vi "BenchC2_DEV_v15_5.vi"() -> ()   [LabVIEW 2017]
uses:
  x64/Debug/BERTTA.dll
panel:
  out "Started:":string
  in  "SHUTDOWN":bool
  in  "MASTER CONTROL":bool
  in  "Tab Control":T1(tab)
  out "Output File":path caption="selected path"
  in  "Browse folder":path=path "" caption="start path"
  in  "Read Seq":bool
  in  "Save Seq":bool
  in  "Configuration file":path caption="Filename"
  in  "OK Button 2":bool
  out "Boolean":bool
  in  "User (initials)":string
  in  "Project name":string
  in  "Description":string
  out "Led11 12":bool
  out "Led11 11":bool
  out "PUMP1":bool
  out "Target amount":dbl format="Target amount:        %#_g"
  out "Scale weight":dbl format="Scale weight:     %#_4g"
  out "Amount now":dbl format="Amount now:      %#_4g"
  out "Flow rate":dbl format="Flow rate:                   %#_4g"
  out "Time to target":dbl format="Time to target:     %<%H:%M:%S>t"
  out "Current step":dbl format="Current step:              %#_g"
  out "Target":dbl format="Target:                %#_4g"
  out "Amount now":dbl format="Amount now:    %#_4g"
  out "Amount now":dbl
  out "Target":dbl
  out "Current step":dbl
  out "Time to target":dbl format="%<%H:%M:%S>t"
  out "Flow rate":dbl
  out "Amount now":dbl
  out "Scale weight":dbl
  out "Target amount":dbl
  out "PUMP2":bool
  out "Sensor OK 6":bool
  out "Sensor OK 5":bool
  out "Sensor OK 4":bool
  out "Sensor OK 3":bool
  in  "OK Button":bool
  in  "Add comment":string
  out "Tr":dbl format="Tr:              %#_4g"
  out "Tj in":dbl format="Tj in:        %#_4g"
  out "Tj out":dbl format="Tj out:        %#_4g"
  out "T set":dbl format="T set:          %#_g"
  out "Current step":i32 format="Current step:  %.0f"
  out "RPM":dbl format="RPM:          %#_g"
  out "Torque 2":dbl format="Torque:      %#_g"
  out "PUMP3":bool
  out "Target amount":dbl
  out "Scale weight":dbl
  out "Amount now":dbl
  out "Flow rate":dbl
  out "Time to target":dbl format="%<%H:%M:%S>t"
  out "Current step":dbl
  out "Target":dbl
  out "Amount now":dbl
  out "Waveform Chart 5":dynamicdata(graph)
  out "Waveform Chart 6":dynamicdata(graph)
  out "Waveform Chart 7":dynamicdata(graph)
  out "Led11 10":bool
  out "T external 3":dbl format="T (S2):       %#_4g"
  out "Table":string[][](table)=[["14.8.2017 18.06.59", "0,000000", "417,670000", "-0,150000", "1,000000", "22,220000", "23,366837", "23,574959", "23,985852", "23,690000", "240,000000", "4,000000", "0,000000", "397,000000", "-397,000000", "1,000000"], ["14.8.2017 18.07.06", "0,000000", "417,640000", "-0,120000", "1,000000", "22,220000", "23,763115", "23,906257", "23,985694", "23,680000", "240,000000", "4,000000", "0,000000", "397,000000", "-397,000000", "1,000000"], ["14.8.2017 18.07.13", "0,000000", "417,640000", "-0,120000", "1,000000", "22,220000", "23,965922", "24,013440", "23,984906", "23,670000", "240,000000", "4,100000", "3,000000", "397,000000", "-397,000000", "1,000000"], ["14.8.2017 18.07.21", "0,000000", "417,640000", "-0,120000", "1,000000", "22,220000", "23,943860", "23,900110", "23,987113", "23,670000", "240,000000", "4,000000", "0,000000", "397,000000", "-397,000000", "1,000000"], ["14.8.2017 18.07.28", "0,000000", "417,640000", "-0,120000", "1,000000", "22,220000", "23,736328", "23,600018", "23,989004", "23,660000", "240,000000", "4,000000", "0,000000", "397,000000", "-397,000000", "1,000000"], ["14.8.2017 18.07.36", "0,000000", "417,640000", "-0,120000", "1,000000", "22,220000", "23,480910", "23,324538", "23,991053", "23,660000", "240,000000", "4,000000", "0,000000", "397,000000", "-397,000000", "1,000000"], ["14.8.2017 18.07.43", "0,000000", "417,640000", "-0,120000", "2,000000", "22,220000", "23,195579", "23,008270", "23,999093", "23,650000", "240,000000", "4,000000", "0,000000", "397,000000", "-397,000000", "1,000000"], ["14.8.2017 18.07.51", "0,000000", "417,650000", "-417,650000", "1,000000", "22,220000", "22,862541", "22,649021", "24,003979", "23,650000", "240,000000", "4,000000", "0,000000", "397,000000", "-397,000000", "2,000000"], ["14.8.2017 18.07.58", "0,000000", "417,640000", "0,010000", "1,000000", "22,220000", "22,541353", "22,354878", "24,005398", "23,650000", "240,000000", "4,000000", "0,000000", "397,000000", "-397,000000", "1,000000"], ["14.8.2017 18.08.06", "0,000000", "417,640000", "0,010000", "1,000000", "22,220000", "22,347931", "22,253738", "24,007605", "23,640000", "240,000000", "4,100000", "0,000000", "397,000000", "-397,000000", "1,000000"], ["14.8.2017 18.08.13", "0,000000", "417,640000", "0,010000", "1,000000", "22,220000", "22,329030", "22,302102", "24,006028", "23,640000", "240,000000", "4,000000", "0,000000", "395,820000", "-395,820000", "1,000000"], ["14.8.2017 18.08.20", "0,000000", "417,640000", "0,010000", "1,000000", "22,220000", "22,466849", "22,511320", "24,002403", "23,630000", "240,000000", "4,000000", "0,000000", "395,830000", "-0,010000", "1,000000"], ["14.8.2017 18.08.28", "0,000000", "417,640000", "0,010000", "1,000000", "22,220000", "22,707062", "22,835101", "24,000984", "23,620000", "240,000000", "4,000000", "0,000000", "395,830000", "-0,010000", "1,000000"], ["14.8.2017 18.08.35", "0,000000", "417,640000", "0,010000", "1,000000", "22,220000", "23,054104", "23,232979", "24,001299", "23,600000", "240,000000", "4,000000", "0,000000", "395,830000", "-0,010000", "1,000000"], ["14.8.2017 18.08.43", "0,000000", "417,640000", "0,010000", "1,000000", "22,220000", "23,412371", "23,522793", "24,002560", "23,590000", "240,000000", "4,000000", "0,000000", "395,820000", "0,000000", "1,000000"], ["14.8.2017 18.08.51", "0,000000", "417,640000", "0,010000", "1,000000", "22,220000", "23,596247", "23,656125", "24,003821", "23,580000", "240,000000", "4,000000", "0,000000", "395,820000", "0,000000", "1,000000"]]
  out "LED_5":bool
  out "LED_4":bool
  in  "PAUSE/RUN 4":bool
  in  "TEMP RAMP":dbl[][](array[numeric])
  out "LED_3":bool
  out "LED_2":bool
  out "LED_1":bool
  out "LED_MANUAL":bool
  in  "Reset 6":bool
  in  "Manual/Ramp":bool=TRUE
  in  "Sensor selector":bool=TRUE
  in  "Tr/Tj mode selector":bool=TRUE
  out "LED STOP":bool
  in  "Failsafe":dbl=20.0 format="Failsafe temperature:            %#_g"
  out "Current temp":dbl format="Current temperature S1:       %#_4g"
  out "Sensor OK":bool
  out "T external 2":dbl format="Current temperature S2:       %#_4g"
  in  "OK Button 3":bool
  out "Waveform Chart":dynamicdata(graph)
  in  "X scale":i64(slide)=50 scale=0.0..100.0
  out "Led11 7":bool
  out "Led11 6":bool
  out "Led11 7":bool
  out "Led11 6":bool
  out "Led5 7":bool
  out "Led4 6":bool
  out "Waveform Chart 18":dynamicdata(graph)
  in  "PAUSE/RUN 3":bool
  in  "Tube select 3":u32(ring) items=["Big tube", "Double big tube", "Medium tube", "Small tube"]
  in  "Reset 8":bool
  out "Led11 9":bool
  in  "?":bool
  in  "Grams / min 3":dbl
  out "RPM 3":dbl format="%_4f"
  out "Flow rate (g/min) 3":dbl
  out "Scale reading 3":dbl
  out "Step amount now 3":dbl
  out "Total amount now 3":dbl
  out "Elapsed / step 3":dbl format="%<%H:%M:%S>t"
  out "Time to target 3":dbl format="%<%H:%M:%S>t"
  out "Led5 5":bool
  out "Led4 5":bool
  out "Led3 5":bool
  out "Led2 5":bool
  out "Led1 5":bool
  in  "PumpSeq 6":dbl[][](array[numeric])=[[0.0, 0.0, 0.0, 0.0, 0.0, 0.0, 0.0, 0.0, 0.0, 0.0], [0.0, 0.0, 0.0, 0.0, 0.0, 0.0, 0.0, 0.0, 0.0, 0.0], [0.0, 0.0, 0.0, 0.0, 0.0, 0.0, 0.0, 0.0, 0.0, 0.0], [0.0, 0.0, 0.0, 0.0, 0.0, 0.0, 0.0, 0.0, 0.0, 0.0], [0.0, 0.0, 0.0, 0.0, 0.0, 0.0, 0.0, 0.0, 0.0, 0.0], [0.0, 0.0, 0.0, 0.0, 0.0, 0.0, 0.0, 0.0, 0.0, 0.0], [0.0, 0.0, 0.0, 0.0, 0.0, 0.0, 0.0, 0.0, 0.0, 0.0], [0.0, 0.0, 0.0, 0.0, 0.0, 0.0, 0.0, 0.0, 0.0, 0.0], [0.0, 0.0, 0.0, 0.0, 0.0, 0.0, 0.0, 0.0, 0.0, 0.0], [0.0, 0.0, 0.0, 0.0, 0.0, 0.0, 0.0, 0.0, 0.0, 0.0]]
  out "Led11 8":bool
  in  "PAUSE/RUN 2":bool
  in  "Tube select 2":u32(ring) items=["Big tube", "Double big tube", "Medium tube", "Small tube"]
  out "Led11 7":bool
  in  "?":bool
  in  "Grams / min 2":dbl
  out "RPM 2":dbl format="%_4f"
  out "Flow rate (g/min) 2":dbl
  out "Scale reading 2":dbl
  out "Step amount now 2":dbl
  out "Total amount now 2":dbl
  out "Elapsed / step 2":dbl format="%<%H:%M:%S>t"
  out "Time to target 2":dbl format="%<%H:%M:%S>t"
  out "Led5 4":bool
  out "Led4 4":bool
  out "Led3 4":bool
  out "Led2 4":bool
  out "Led1 4":bool
  in  "PumpSeq 5":dbl[][](array[numeric])=[[0.0, 0.0, 0.0, 0.0, 0.0, 0.0, 0.0, 0.0, 0.0, 0.0], [0.0, 0.0, 0.0, 0.0, 0.0, 0.0, 0.0, 0.0, 0.0, 0.0], [0.0, 0.0, 0.0, 0.0, 0.0, 0.0, 0.0, 0.0, 0.0, 0.0], [0.0, 0.0, 0.0, 0.0, 0.0, 0.0, 0.0, 0.0, 0.0, 0.0], [0.0, 0.0, 0.0, 0.0, 0.0, 0.0, 0.0, 0.0, 0.0, 0.0], [0.0, 0.0, 0.0, 0.0, 0.0, 0.0, 0.0, 0.0, 0.0, 0.0], [0.0, 0.0, 0.0, 0.0, 0.0, 0.0, 0.0, 0.0, 0.0, 0.0], [0.0, 0.0, 0.0, 0.0, 0.0, 0.0, 0.0, 0.0, 0.0, 0.0], [0.0, 0.0, 0.0, 0.0, 0.0, 0.0, 0.0, 0.0, 0.0, 0.0], [0.0, 0.0, 0.0, 0.0, 0.0, 0.0, 0.0, 0.0, 0.0, 0.0]]
  out "Led11 6":bool
  in  "Reset 7":bool
  in  "PAUSE/RUN":bool
  in  "Tube select":u32(ring) items=["Big tube", "Double big tube", "Medium tube", "Small tube"]
  out "Led11 5":bool
  out "RPM":dbl format="RPM                      %_4f"
  out "Flow rate (g/min)":dbl format="Flow rate               %#_g"
  out "Scale reading":dbl format="Scale reading       %#_g"
  out "Step amount now":dbl format="Step amount       %#_g"
  out "Total amount now":dbl format="Total amount      %#_g"
  out "Elapsed / step":dbl format="Elapsed / step      %<%H:%M:%S>t"
  out "Time to target":dbl format="Time to target     %<%H:%M:%S>t"
  out "Led5 3":bool
  out "Led4 3":bool
  out "Led3 3":bool
  out "Led2 3":bool
  out "Led1 3":bool
  in  "PumpSeq 4":dbl[][](array[numeric])=[[0.0, 0.0, 0.0, 0.0, 0.0, 0.0, 0.0, 0.0, 0.0, 0.0], [0.0, 0.0, 0.0, 0.0, 0.0, 0.0, 0.0, 0.0, 0.0, 0.0], [0.0, 0.0, 0.0, 0.0, 0.0, 0.0, 0.0, 0.0, 0.0, 0.0], [0.0, 0.0, 0.0, 0.0, 0.0, 0.0, 0.0, 0.0, 0.0, 0.0], [0.0, 0.0, 0.0, 0.0, 0.0, 0.0, 0.0, 0.0, 0.0, 0.0], [0.0, 0.0, 0.0, 0.0, 0.0, 0.0, 0.0, 0.0, 0.0, 0.0], [0.0, 0.0, 0.0, 0.0, 0.0, 0.0, 0.0, 0.0, 0.0, 0.0], [0.0, 0.0, 0.0, 0.0, 0.0, 0.0, 0.0, 0.0, 0.0, 0.0], [0.0, 0.0, 0.0, 0.0, 0.0, 0.0, 0.0, 0.0, 0.0, 0.0], [0.0, 0.0, 0.0, 0.0, 0.0, 0.0, 0.0, 0.0, 0.0, 0.0]]
  in  "?":bool
  in  "Grams / min":dbl format="Manual g/min:  %#_g"
  out "Led11 4":bool
  in  "Reset 5":bool
  in  "OK Button 4":bool
  out "Waveform Chart 16":dynamicdata(graph)
  in  "OK Button 5":bool
  out "Waveform Chart 17":dynamicdata(graph)
  in  "OK Button 6":bool
  in  "PAUSE/RUN 5":bool
  in  "?":bool
  in  "Scale port":dbl=5.0
  out "Waveform Chart 15":dynamicdata(graph)
  in  "OK Button 8":bool
  in  "PAUSE/RUN 6":bool
  in  "Set RPM":i32
  in  "Remote / Manual":bool
  out "RPM":dbl
  out "Torque":dbl
  out "Waveform Chart 4":dynamicdata(graph)
  in  "OK Button 7":bool
  in  "CDAQ Temp Control":tag="cDAQ9188XT-1C3BF12Mod1"
  in  "CDAQ PAM Control":tag="cDAQ9188XT-1C3BF12Mod1"
  in  "PORT PUMP2":i32 format="PUMP 2 PORT:  %.0f"
  in  "PORT PUMP3":i32 format="PUMP 3 PORT:  %.0f"
  in  "PORT PUMP1":i32 format="PUMP 1 PORT:  %.0f"
  in  "Save PortDev":bool
  in  "LAUDA":i32 format="LAUDA PORT:  %.0f"
  in  "HEIDOLPH":i32 format="HEIDOLPH PORT:  %.0f"
  in  "SCALE1":i32 format="SCALE 1 PORT:  %.0f"
  in  "SCALE2":i32 format="SCALE 2 PORT:  %.0f"
  in  "SCALE 3":i32 format="SCALE 3 PORT:  %.0f"
  # "PUMP & SCALE 1"
  # "PUMP & SCALE 2"
  # "PUMP & SCALE 3"
  # "STEP"
  # "STEP"
  # "STEP"
  # "TOTAL"
  # "TOTAL"
  # "TOTAL"
  # "Temperature sensor:"
  # "Manual control:"
  # "MANUAL"
  # "RAMP"
  # "Temp Target       Time Target          Wait Time"
  # "STOP"
  # "g              min"
  # "g              min"
  # "g              min"
  # "PAM control"
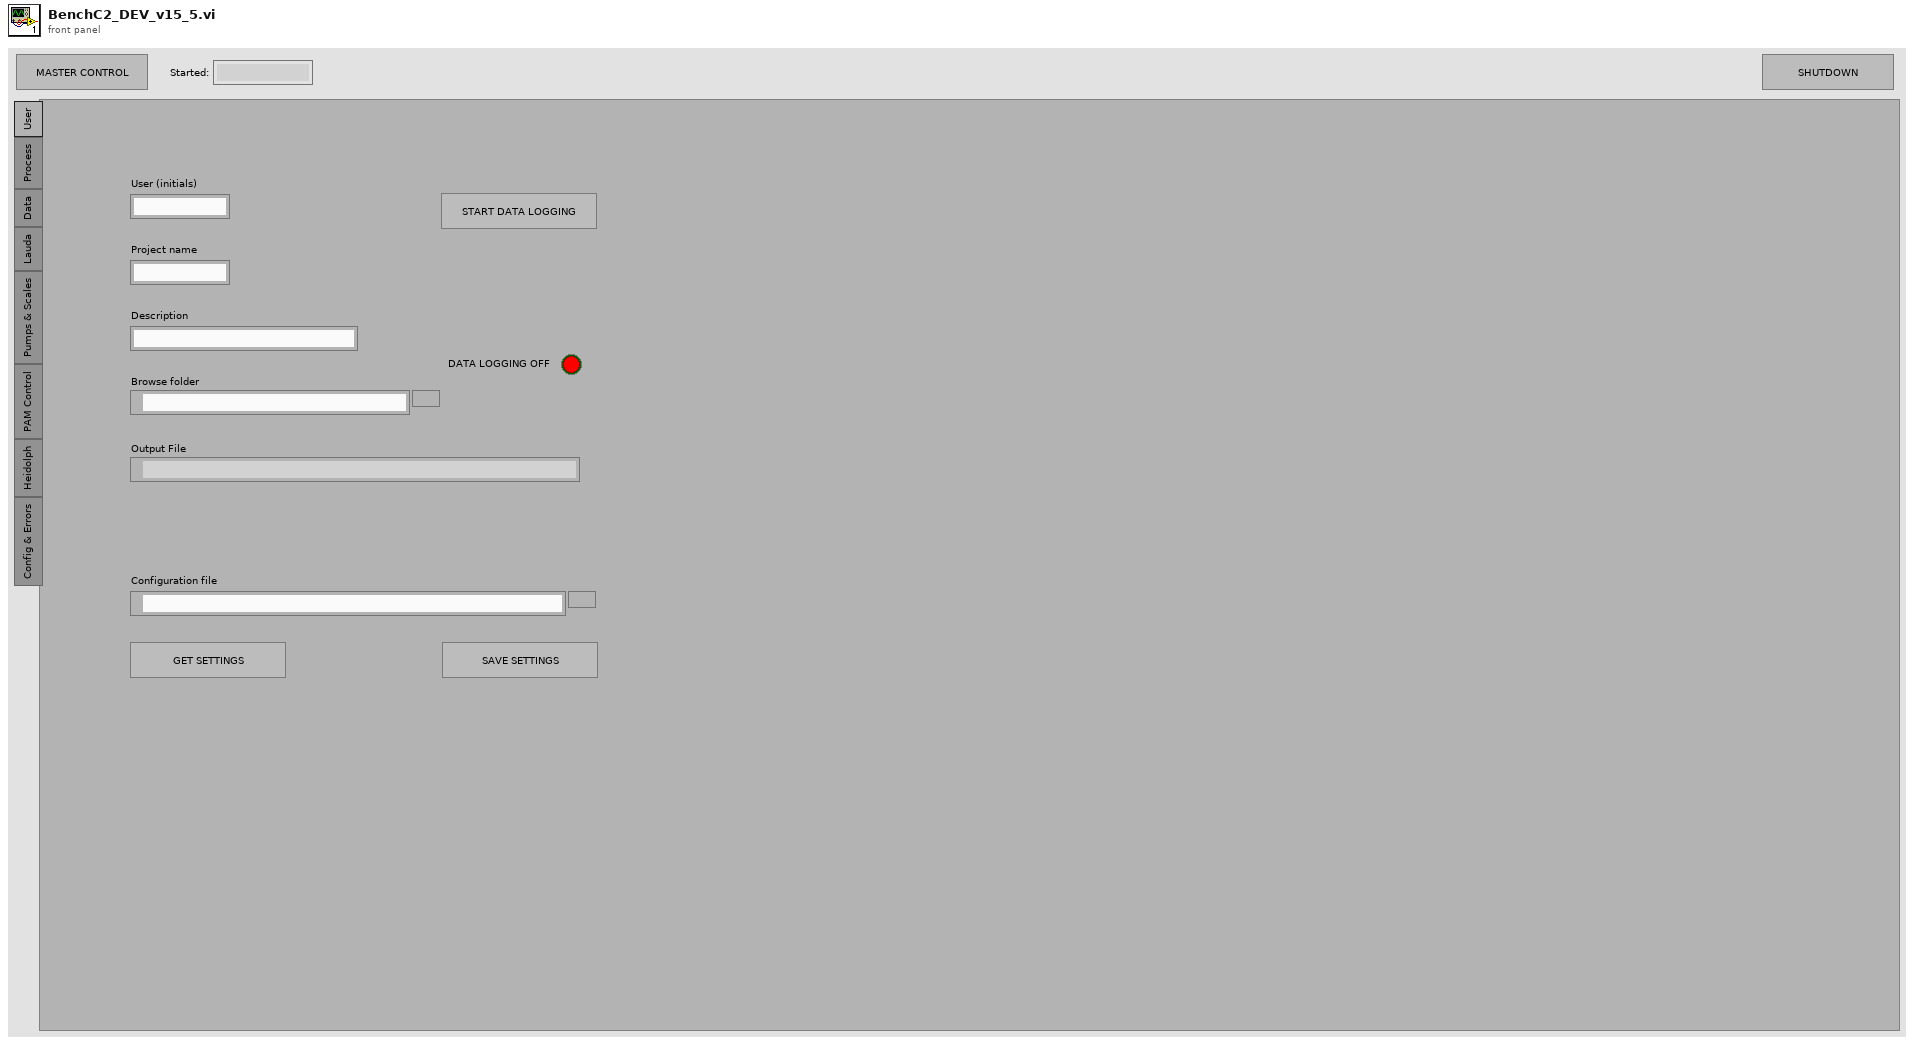
[diagram p1: front panel]
types:
  T1 = enum32{"User", "Process", "Data", "Lauda", "Pumps & Scales", "PAM Control", "Heidolph", "Config & Errors"}
diagram:
  n1 = while {
    i -> [w217]
    stop <- FALSE stop-if-true
    w49 = i64 1000 ("y")
    # "TARKISTA: negatiiviset lämpötilat, toimivatko"
    # "X-skaalaus puuttuu"
    # "SCALE & PUMP 1"
    # "SCALE & PUMP 3"
    n2 = And(x="PAUSE/RUN 6", y="MASTER CONTROL") -> (x .and. y?=w30:bool)
    n3 = feedback #1() -> (w54:dbl[][])  [unwired: 1 in]
    n4 = Select(t="TEMP RAMP", s="Reset 6", f=w54) -> (s? t:f=w55:dbl[][])
    n5 = feedback-in #1(w55) -> ()
    n6 = Initialize Array(0.0 ("element"), 5 ("dimension size"), 3 ("dimension size")) -> (w98:dbl[][])
    n7 = Select(t="Set RPM", s=w30, f=10) -> (s? t:f=w33:i32)
    n8 = Not(x="MASTER CONTROL") -> (.not. x?=w266:bool)
    n9 = Replace Array Subset(array=w98, new element=w54, index (row)=0, index (col)=0 ("disabled index (col)")) -> (w72:dbl[][])
    n10 = control-ref of="This VI"() -> (w26:refnum<vi>)
    n11 = Multiply(x="X scale", y=w49) -> (x*y=w50:i64)
    n12 = Boolean To (0,1)(Boolean=w266) -> (0, 1=w267:i16)
    n13 = Add(x=w50, y=w49) -> (x+y=w45:i64)
    n14 = for {
      N: w267 -> [_]
      n15 = Get Date/Time String(want seconds? (F)=TRUE) -> (time string=→"Started:":string)  [unwired: 2 in, 1 out]
    }
    n16 = feedback #2() -> (w48:i64)  [unwired: 1 in]
    n17 = feedback-in #2(w45) -> ()
    n18 = Boolean To (0,1)(Boolean="Sensor selector") -> (0, 1=w80:i16)
    n19 = Boolean To (0,1)(Boolean="SHUTDOWN") -> (0, 1=w24:i16)
    n20 = call "shutdown sequence.vi"("SHUTDOWN"="SHUTDOWN", "VI in"=w26) -> ()  [unwired: 10 in]
    n21 = Not Equal?(x=w48, y=w45) -> (x != y?=w47:bool)
    n22 = property on="Waveform Chart" class="WFChart (strict)"() -> ("History Data"=w52:dynamicdata[])  [unwired: 2 in, 2 out]
    n23 = Boolean To (0,1)(Boolean=w47) -> (0, 1=w44:i16)
    n24 = Array Size(array=w52) -> (size(s)=w46:i32)
    n25 = Boolean To (0,1)(Boolean="SHUTDOWN") -> (0, 1=w27:i16)
    n26 = Boolean To (0,1)(Boolean="Tr/Tj mode selector") -> (0, 1=w92:i16)
    n27 = formula code="int SensorLED1 = 0, SensorLED0 = 0, ModeLED1 = 0, ModeLED0 = 0;\nif(Sensor==1) SensorLED1 = 1;\nif(Sensor==0) SensorLED0 = 1;\nif(Tr_Tj==1) ModeLED1 = 1;\nif(Tr_Tj==0) ModeLED0 = 1;"("Tr_Tj"=w92, "Sensor"=w80) -> ("SensorLED1"=w90:i32, "SensorLED0"=w88:i32, "ModeLED1"=w73:i32, "ModeLED0"=w83:i32)
    n28 = Equal?(x=w90, y=1.0) -> (x = y?=→"Sensor OK 3":bool)
    n29 = Equal?(x=w88, y=1.0) -> (x = y?=→"Sensor OK 4":bool)
    n30 = for {
      N: w44 -> [_]
      tunnel: w46 -> [w274]
      tunnel: w45 -> [w273]
      n31 = Add(x=w274, y=w273) -> (x+y=w272:i64)
      n32 = property on="Waveform Chart" class="WFChart (strict)"("XScale.Maximum"=w272) -> ()  [unwired: 2 in, 2 out]
    }
    n33 = call "MReadRS232_2.vi"("port1"="LAUDA", "dev1"=1, "port2"="LAUDA", "dev2"=2, "port3"="HEIDOLPH", "dev7"=5, "dev8"=0, "port7"="SCALE 3", "port8"=0, "dev5"=5, "port5"="SCALE1", "dev4"=4, "dev6"=5, "port6"="SCALE2", "port4"="HEIDOLPH", "dev3"=3) -> ("params"=w1:dbl[])  [unwired: 2 in, 1 out]
    n34 = call "HEI_CTRL.vi"("shutdown"=w27, "Set RPM"=w33, "Remote / Manual"="Remote / Manual", "port3"="HEIDOLPH") -> ()  [unwired: 8 in]
    n35 = And(x="MASTER CONTROL", y="PAUSE/RUN 4") -> (x .and. y?=w116:bool)
    n36 = Index Array(array=w72, index (col)=2 ("disabled index (col)")) -> (element=w104:dbl[])  [unwired: 1 in]
    n37 = Equal?(x=w73, y=1.0) -> (x = y?=→"Sensor OK 6":bool)
    n38 = Equal?(x=w83, y=1.0) -> (x = y?=→"Sensor OK 5":bool)
    n39 = Boolean To (0,1)(Boolean=w116) -> (0, 1=w115:i16)
    n40 = Boolean To (0,1)(Boolean="Manual/Ramp") -> (0, 1=w117:i16)
    n41 = Boolean To (0,1)(Boolean="Reset 6") -> (0, 1=w119:i16)
    n42 = Build Array("LAUDA", "HEIDOLPH", "SCALE1", "SCALE2", "SCALE 3", "PORT PUMP1", "PORT PUMP2", "PORT PUMP3") -> (w59:i32[])
    n43 = Index Array(array=w72, index (col)=1 ("disabled index (col)")) -> (element=w106:dbl[])  [unwired: 1 in]
    n44 = Index Array(array=w72, index (col)=0 ("disabled index (col)")) -> (element=w107:dbl[])  [unwired: 1 in]
    n45 = call "LaudaDAQ.vi"("device name"="CDAQ Temp Control") -> (1:"Tj out"=→"Tj out":dbl, "data"=w254:dynamicdata, "Sensor OK"=→"Sensor OK":bool, 4:"Tj out"=→"Tj in":dbl, "T external 2"=w29:dbl)  [unwired: 5 in, 1 out]
    "T external 2" <- w29
    "T external 3" <- w29
    n46 = call "Ramp_Lauda_v3.vi"("manual"=w117, "Tr_Tj"=w92, "shutdown"=w24, "S1_S2"=w80, "Tr"=w1, "T_fail"="Failsafe", "enable"=w115, "time_set"=w106, "reset"=w119, "time_wait"=w104, "T_S2"=w29, "port"="LAUDA", "T_sp"=w107) -> ("LED_1"=→"LED_1":bool, "LED_manual"=→"LED_MANUAL":bool, "LED_2"=→"LED_2":bool, "step"=w70:dbl, "LED_stop"=→"LED STOP":bool, "LED_3"=→"LED_3":bool, "LED 4"=→"LED_4":bool, "LED 5"=→"LED_5":bool, "setpoint"=w67:dbl, "Tr_out"=w114:dbl, "T int"=w113:dbl)  [unwired: 2 in, 2 out]
    "Tr" <- w114
    "T set" <- w67
    "Current temp" <- w114
    n47 = Boolean To (0,1)(Boolean="Save PortDev") -> (0, 1=w220:i16)
    n48 = for {
      N: w220 -> [_]
      tunnel: w59 -> [w320]
      tunnel: "Save PortDev" -> [w321]
      n49 = call "Convert to Dynamic Data"("Array"=w320) -> ("Dynamic Data Type"=w319:dynamicdata)  [unwired: 3 in]
      n50 = call "Write To Measurement File3"("Signals"=w319, "Reset"=w321) -> ()  [unwired: 15 in, 3 out]
    }
    n51 = Add(x=w70, y=1.0) -> (x+y=→"Current step":dbl)
    n52 = Less?(x=w217, y=1.0) -> (x < y?=w215:bool)
    n53 = Index Array(array=w1, index=3) -> (element=w208:dbl)
    "RPM" <- w208
    "RPM" <- w208
    n54 = Index Array(array=w1, index=2) -> (element=w210:dbl)
    n55 = Boolean To (0,1)(Boolean=w215) -> (0, 1=w216:i16)
    n56 = Divide(x=w210, y=10.0) -> (x/y=w207:dbl)
    "Torque" <- w207
    "Torque 2" <- w207
    n57 = for {
      N: w216 -> [_]
      tunnel: w215 -> [w314]
      n58 = while {
        tunnel: [w317] -> w313
        tunnel: w314 -> [w315]
        stop <- w318 stop-if-true
        n59 = call "Read From Measurement File2"("Enable"=TRUE, "Reset"=w315) -> ("Signals"=w317:dynamicdata, "EOF?"=w318:bool)  [unwired: 4 in, 4 out]
      }
      n60 = call "Convert from Dynamic Data2"("Dynamic Data Type"=w313) -> ("Array"=w299:dbl[])  [unwired: 3 in]
      n61 = Index Array(array=w299, index=0) -> (element=w306:dbl)
      n62 = Index Array(array=w299, index=1) -> (element=w305:dbl)
      n63 = Index Array(array=w299, index=2) -> (element=w304:dbl)
      n64 = Index Array(array=w299, index=3) -> (element=w303:dbl)
      n65 = Index Array(array=w299, index=4) -> (element=w302:dbl)
      n66 = Index Array(array=w299, index=5) -> (element=w296:dbl)
      n67 = Index Array(array=w299, index=6) -> (element=w298:dbl)
      n68 = Index Array(array=w299, index=7) -> (element=w297:dbl)
      n69 = property on="LAUDA" class="DigNum (strict)"("Val(Sgnl)"=w306) -> ()  [unwired: 2 in, 2 out]
      n70 = property on="HEIDOLPH" class="DigNum (strict)"("Val(Sgnl)"=w305) -> ()  [unwired: 2 in, 2 out]
      n71 = property on="SCALE1" class="DigNum (strict)"("Val(Sgnl)"=w304) -> ()  [unwired: 2 in, 2 out]
      n72 = property on="SCALE2" class="DigNum (strict)"("Val(Sgnl)"=w303) -> ()  [unwired: 2 in, 2 out]
      n73 = property on="SCALE 3" class="DigNum (strict)"("Val(Sgnl)"=w302) -> ()  [unwired: 2 in, 2 out]
      n74 = property on="PORT PUMP2" class="DigNum (strict)"("Val(Sgnl)"=w298) -> ()  [unwired: 2 in, 2 out]
      n75 = property on="PORT PUMP3" class="DigNum (strict)"("Val(Sgnl)"=w297) -> ()  [unwired: 2 in, 2 out]
      n76 = property on="PORT PUMP1" class="DigNum (strict)"("Val(Sgnl)"=w296) -> ()  [unwired: 2 in, 2 out]
    }
    n77 = Merge Signals(w208, w207) -> (w206:dynamicdata)
    "Waveform Chart 4" <- w206
    "Waveform Chart 6" <- w206
    n78 = Boolean To (0,1)(Boolean="OK Button 3") -> (0, 1=w235:i16)
    n79 = for {
      N: w235 -> [_]
      n80 = property on="Waveform Chart" class="WFChart (strict)"("History Data"=dynamicdata[] []) -> ()  [unwired: 2 in, 2 out]
    }
    n81 = Merge Signals(w67, w114, w113, w254) -> (w255:dynamicdata)
    "Waveform Chart" <- w255
    "Waveform Chart 5" <- w255
    n82 = Boolean To (0,1)(Boolean="OK Button 4") -> (0, 1=w233:i16)
    n83 = for {
      N: w233 -> [_]
      n84 = property on="Waveform Chart 18" class="WFChart (strict)"("History Data"=dynamicdata[] []) -> ()  [unwired: 2 in, 2 out]
    }
    n85 = Boolean To (0,1)(Boolean="OK Button 5") -> (0, 1=w78:i16)
    n86 = call "IsmaCTRL.vi"("FR_manual"="Grams / min", "Manual"="?", "Reset"="Reset 5", "Pause"="PAUSE/RUN", "Setpoint_W   /   Setpoint_T"="PumpSeq 4", "Enable"="MASTER CONTROL", "Scale"=w1) -> ("Boolean 9"=→"Led11 5" →"Led11 10":bool, "Boolean"=→"Led1 3":bool, "Boolean 2"=→"Led2 3":bool, "Boolean 3"=→"Led3 3":bool, "Boolean 4"=→"Led4 3":bool, "Boolean 5"=→"Led5 3":bool, "Boolean 6"=→"Led4 6":bool, "Boolean 7"=→"Led5 7":bool, "FR"=w6:dbl, "RPM"=w5:dbl, "Weight"=w4:dbl, "elapsed"=→"Elapsed / step":dbl, "time_to_target"=→"Time to target" →"Time to target":dbl, "pumpCTRL"=w18:dbl, "Boolean 8"=w10:bool)  [unwired: 6 in]
    "Flow rate" <- w6
    "Scale weight" <- w4
    "Led11 4" <- w10
    "Scale reading" <- w4
    "Flow rate (g/min)" <- w6
    "RPM" <- w5
    n87 = for {
      N: w78 -> [_]
      n88 = property on="Waveform Chart 16" class="WFChart (strict)"("History Data"=dynamicdata[] []) -> ()  [unwired: 2 in, 2 out]
    }
    n89 = Greater?(x=w18, y=70.0) -> (0:→"PUMP1":bool)
    n90 = Merge Signals(w4, w6) -> (w79:dynamicdata)
    "Waveform Chart 18" <- w79
    n91 = Multiply(x=-1.0, y=w4) -> (x*y=→"Amount now" →"Total amount now":dbl)
    n92 = Boolean To (0,1)(Boolean="OK Button 6") -> (0, 1=w76:i16)
    n93 = for {
      N: w76 -> [_]
      n94 = property on="Waveform Chart 17" class="WFChart (strict)"("History Data"=dynamicdata[] []) -> ()  [unwired: 2 in, 2 out]
    }
    n95 = And(x="PAUSE/RUN", y=w10) -> (x .and. y?=w194:bool)
    n96 = feedback #3() -> (w195:bool)  [unwired: 1 in]
    n97 = feedback-in #3(w194) -> ()
    n98 = Not Equal?(x=w195, y=w194) -> (x != y?=w193:bool)
    n99 = Boolean To (0,1)(Boolean=w193) -> (0, 1=w192:i16)
    n100 = for {
      N: w192 -> [_]
      n101 = property on="PAUSE/RUN" class="Bool (strict)"("Val(Sgnl)"=FALSE ("Value (Signaling)")) -> ()  [unwired: 2 in, 2 out]
    }
    n102 = Boolean To (0,1)(Boolean="OK Button 7") -> (0, 1=w231:i16)
    n103 = for {
      N: w231 -> [_]
      n104 = property on="Waveform Chart 4" class="WFChart (strict)"("History Data"=dynamicdata[] []) -> ()  [unwired: 2 in, 2 out]
    }
    n105 = Boolean To (0,1)(Boolean="OK Button 8") -> (0, 1=w203:i16)
    n106 = for {
      N: w203 -> [_]
      n107 = property on="Waveform Chart 15" class="WFChart (strict)"("History Data"=dynamicdata[] []) -> ()  [unwired: 2 in, 2 out]
    }
    n108 = Index Array(array="PumpSeq 5", index (col)=0) -> (element=w175:dbl[])  [unwired: 1 in]
    n109 = Index Array(array="PumpSeq 5", index (col)=1) -> (element=w176:dbl[])  [unwired: 1 in]
    n110 = Boolean To (0,1)(Boolean="PAUSE/RUN 2") -> (0, 1=w190:i16)
    n111 = Boolean To (0,1)(Boolean="MASTER CONTROL") -> (0, 1=w191:i16)
    n112 = And(x=w191, y=w190) -> (x .and. y?=w189:i16)
    n113 = Boolean To (0,1)(Boolean="Reset 7") -> (0, 1=w180:i16)
    n114 = Boolean To (0,1)(Boolean="?") -> (0, 1=w182:i16)
    n115 = call "PID_Flow Ctrl_2 P2.vi"("weight"=w1, "Setpoint_W"=w175, "Setpoint_T"=w176, "FrManual"="Grams / min 2", "enable"=w189, "manual"=w182, "reset"=w180, "tube"="Tube select 2") -> ("elapsed_step"=→"Elapsed / step 2":dbl, "total_target"=→"Target":dbl, "Setpoint_W"=→"Target amount":dbl, "LED_stop"=w158:bool, "RPM"=w163:dbl, "LED1"=→"Led1 4":bool, "LED4"=→"Led4 4":bool, "LED2"=→"Led2 4":bool, "step_amount"=→"Amount now" →"Step amount now 2":dbl, "LED3"=→"Led3 4":bool, "LED5"=→"Led5 4":bool, "weight"=w127:dbl, "time_to_target"=→"Time to target" →"Time to target 2":dbl, "LED6"=→"Led11 6":bool, "LED7"=→"Led11 7":bool, "PumpCTRL"=w166:dbl, "step"=→"Current step":dbl, "LED_manual"=→"Led11 7" →"Led11 11":bool, "FR"=w164:dbl)  [unwired: 1 in]
    "Scale weight" <- w127
    "Flow rate" <- w164
    "Led11 6" <- w158
    "Scale reading 2" <- w127
    "Flow rate (g/min) 2" <- w164
    "RPM 2" <- w163
    n116 = Merge Signals(w127, w164) -> (w165:dynamicdata)
    "Waveform Chart 16" <- w165
    n117 = Multiply(x=w127, y=-1.0) -> (x*y=→"Amount now" →"Total amount now 2":dbl)
    n118 = And(x="PAUSE/RUN 2", y=w158) -> (x .and. y?=w161:bool)
    n119 = Greater?(x=w166, y=70.0) -> (0:→"PUMP2":bool)
    n120 = feedback #4() -> (w162:bool)  [unwired: 1 in]
    n121 = feedback-in #4(w161) -> ()
    n122 = Not Equal?(x=w162, y=w161) -> (x != y?=w160:bool)
    n123 = Boolean To (0,1)(Boolean=w160) -> (0, 1=w159:i16)
    n124 = for {
      N: w159 -> [_]
      n125 = property on="PAUSE/RUN 2" class="Bool (strict)"("Val(Sgnl)"=FALSE ("Value (Signaling)")) -> ()  [unwired: 2 in, 2 out]
    }
    n126 = Index Array(array="PumpSeq 6", index (col)=0) -> (element=w144:dbl[])  [unwired: 1 in]
    n127 = Index Array(array="PumpSeq 6", index (col)=1) -> (element=w145:dbl[])  [unwired: 1 in]
    n128 = Boolean To (0,1)(Boolean="MASTER CONTROL") -> (0, 1=w152:i16)
    n129 = Boolean To (0,1)(Boolean="PAUSE/RUN 3") -> (0, 1=w151:i16)
    n130 = And(x=w152, y=w151) -> (x .and. y?=w150:i16)
    n131 = Boolean To (0,1)(Boolean="?") -> (0, 1=w143:i16)
    n132 = Boolean To (0,1)(Boolean="Reset 8") -> (0, 1=w141:i16)
    n133 = call "PID_Flow Ctrl_2 P3.vi"("weight"=w1, "Setpoint_W"=w144, "Setpoint_T"=w145, "FrManual"="Grams / min 3", "enable"=w150, "manual"=w143, "reset"=w141, "tube"="Tube select 3") -> ("elapsed_step"=→"Elapsed / step 3":dbl, "total_target"=→"Target":dbl, "Setpoint_W"=→"Target amount":dbl, "LED_stop"=w120:bool, "RPM"=w125:dbl, "LED1"=→"Led1 5":bool, "LED4"=→"Led4 5":bool, "LED2"=→"Led2 5":bool, "step_amount"=→"Amount now" →"Step amount now 3":dbl, "LED3"=→"Led3 5":bool, "LED5"=→"Led5 5":bool, "weight"=w126:dbl, "time_to_target"=→"Time to target" →"Time to target 3":dbl, "LED6"=→"Led11 6":bool, "LED7"=→"Led11 7":bool, "PumpCTRL"=w138:dbl, "step"=→"Current step":dbl, "LED_manual"=→"Led11 9" →"Led11 12":bool, "FR"=w131:dbl)  [unwired: 1 in]
    "Scale weight" <- w126
    "Flow rate" <- w131
    "Led11 8" <- w120
    "Scale reading 3" <- w126
    "Flow rate (g/min) 3" <- w131
    "RPM 3" <- w125
    n134 = call "MWriteRS232_1.vi"("PORT PUMP3"="PORT PUMP3", "PORT PUMP2"="PORT PUMP2", "PORT PUMP1"="PORT PUMP1", "PORT LAUDA"="LAUDA", "P3"=w125, "P2"=w163, "P1"=w5, "LAUDA"=w67) -> ()  [unwired: 4 in]
    n135 = call "Convert to Dynamic Data4"("2D Array"="PumpSeq 6") -> ("Dynamic Data Type"=w241:dynamicdata)  [unwired: 3 in]
    n136 = call "Convert to Dynamic Data3"("2D Array"="PumpSeq 5") -> ("Dynamic Data Type"=w242:dynamicdata)  [unwired: 3 in]
    n137 = call "Convert to Dynamic Data2"("2D Array"="PumpSeq 4") -> ("Dynamic Data Type"=w244:dynamicdata)  [unwired: 3 in]
    n138 = Merge Signals(w241, w242, w244) -> (w243:dynamicdata)
    n139 = Greater?(x=w138, y=70.0) -> (0:→"PUMP3":bool)
    n140 = Merge Signals(w126, w131) -> (w130:dynamicdata)
    "Waveform Chart 17" <- w130
    n141 = Boolean To (0,1)(Boolean="Save Seq") -> (0, 1=w240:i16)
    n142 = Multiply(x=w126, y=-1.0) -> (x*y=→"Amount now" →"Total amount now 3":dbl)
    n143 = for {
      N: w240 -> [_]
      tunnel: w243 -> [w362]
      tunnel: "Configuration file" -> [w363]
      tunnel: "Save Seq" -> [w361]
      n144 = call "Write To Measurement File2"("Signals"=w362, "Reset"=w361, "Filename"=w363) -> ()  [unwired: 14 in, 3 out]
    }
    n145 = Merge Signals(w79, w165, w130) -> (w256:dynamicdata)
    n146 = Merge Signals(w4, w127, w126) -> (→"Waveform Chart 7":dynamicdata)
    n147 = And(x="MASTER CONTROL", y=w120) -> (x .and. y?=w123:bool)
    n148 = feedback #5() -> (w124:bool)  [unwired: 1 in]
    n149 = feedback-in #5(w123) -> ()
    n150 = Not Equal?(x=w124, y=w123) -> (x != y?=w122:bool)
    n151 = Boolean To (0,1)(Boolean="Read Seq") -> (0, 1=w239:i16)
    n152 = for {
      N: w239 -> [_]
      tunnel: "Configuration file" -> [w336]
      tunnel: "Read Seq" -> [w335]
      n153 = while {
        tunnel: [w360] -> w356
        tunnel: w336 -> [w359]
        tunnel: w335 -> [w357]
        stop <- w358 stop-if-true
        n154 = call "Read From Measurement File"("Filename"=w359, "Reset"=w357) -> ("Signals"=w360:dynamicdata, "EOF?"=w358:bool)  [unwired: 4 in, 4 out]
      }
      n155 = call "Convert from Dynamic Data"("Dynamic Data Type"=w356) -> ("Array"=w348:dbl[][])  [unwired: 3 in]
      n156 = Array Subset(array=w348, index (row)=20 ("index"), length (row)=10 ("length")) -> (w353:dbl[][])  [unwired: 2 in]
      n157 = Array Subset(array=w348, index (row)=10 ("index"), length (row)=10 ("length")) -> ()  [unwired: 2 in, 1 out]
      n158 = Array Subset(array=w348, index (row)=0 ("index"), length (row)=10 ("length")) -> ()  [unwired: 2 in, 1 out]
      n159 = Array Subset(array=w348, index (row)=30 ("index"), length (row)=8 ("length")) -> (w337:dbl[][])  [unwired: 2 in]
      n160 = property on="PumpSeq 4" class="Arr (strict)"("Val(Sgnl)"=w353) -> ()  [unwired: 2 in, 2 out]
      n161 = Index Array(array=w337, index (row)=2, index (col)=0 ("disabled index (col)")) -> ()  [unwired: 1 out]
      n162 = Index Array(array=w337, index (row)=4, index (col)=0 ("disabled index (col)")) -> ()  [unwired: 1 out]
      n163 = Index Array(array=w337, index (row)=0, index (col)=1 ("disabled index (col)")) -> ()  [unwired: 1 out]
      n164 = Index Array(array=w337, index (row)=1, index (col)=1 ("disabled index (col)")) -> ()  [unwired: 1 out]
    }
    n165 = Boolean To (0,1)(Boolean=w122) -> (0, 1=w121:i16)
    n166 = for {
      N: w121 -> [_]
      n167 = property on="PAUSE/RUN 3" class="Bool (strict)"("Val(Sgnl)"=FALSE ("Value (Signaling)")) -> ()  [unwired: 2 in, 2 out]
    }
    n168 = Merge Signals(w255, w256, w206) -> (w213:dynamicdata)
    n169 = call "Build Table"("Include time data"=TRUE, "Signals"=w213) -> ("Table"=w263:string[][])  [unwired: 3 in, 6 out]
    n170 = Boolean To (0,1)(Boolean="PAUSE/RUN 5") -> (0, 1=w94:i16)
    n171 = for {
      N: w94 -> [_]
      tunnel: "MASTER CONTROL" -> [w278]
      tunnel: "PAUSE/RUN 5" -> [w277]
      n172 = And(x=w277, y="?") -> (x .and. y?=w286:bool)
      n173 = dll-call lib="C:/Users/shresplab/OneDrive - Kemira Oyj/Documents/GitHub/Bertta/BERTTA/x64/Debug/BERTTA.dll" fn="mettler"("port"="Scale port", "msg"=1) -> ("return type"=w280:dbl)  [unwired: 5 in, 2 out]
      n174 = And(x=w278, y=w286) -> (x .and. y?=w283:bool)
      n175 = Initialize Array(FALSE, 1 ("dimension size")) -> (w285:bool[])
      n176 = Replace Array Subset(array=w285, new element=w283, index=0) -> (w282:bool[])
      n177 = call "Convert to Dynamic Data5"("Double"=w280) -> ("Dynamic Data Type"=→"Waveform Chart 15":dynamicdata)  [unwired: 3 in]
      n178 = call "DAQ Assistant"("data"=w282, "device name"="CDAQ PAM Control") -> ()  [unwired: 16 in, 2 out]
    }
    n179 = Delete From Array(array=w263, length=13, index (col)=0 ("index (row)")) -> (array with subset deleted=→"Table":string[][])  [unwired: 1 in, 1 out]
    n180 = call "filenameparser_09.vi"("Description"="Description", "start path"="Browse folder", "Project name"="Project name", "User (initials)"="User (initials)", "OK Button in"="OK Button 2") -> ("appended path 2"=w229:path, "appended path"=w259:path)  [unwired: 4 in, 1 out]
    "Output File" <- w229
    n181 = Boolean To (0,1)(Boolean="OK Button") -> (0, 1=w258:i16)
    n182 = for {
      N: w258 -> [_]
      tunnel: w259 -> [w327]
      w331 = " " ("string")
      n183 = property on="Add comment" class="Str"("Val(Sgnl)"="" ("Value (Signaling)")) -> ()  [unwired: 2 in, 2 out]
      n184 = Get Date/Time String(want seconds? (F)=TRUE) -> (date string=w334:string, time string=w332:string)  [unwired: 2 in]
      n185 = Concatenate Strings(w334, w331, w332, w331, "Add comment") -> (w330:string)
      n186 = feedback #6() -> (w329:string[])  [unwired: 1 in]
      n187 = Build Array (concatenate)(w329, w330) -> (w328:string[])
      n188 = feedback-in #6(w328) -> ()
      n189 = Write to Text File(file (use dialog)=w327, text=w328) -> ()  [unwired: 2 in, 3 out]
    }
    n190 = call "Header Names 4.vi"("Dynamic Data"=w213) -> ("Signals Out"=w214:dynamicdata)  [unwired: 10 in]
    n191 = call "Write To Measurement File"("Signals"=w214, "Enable"="OK Button 2", "Filename"=w229) -> ()  [unwired: 14 in, 3 out]
    "Boolean" <- "OK Button 2"
  }
